vi "save_to_disk.vi"(3 "Retrace":i16[][](array[numeric]), 4 "slice":i32, 5 "write info file?":bool, 6 "error in":errorcluster, 7 "Scan info":string, 8 "Image":i16[][](array[numeric]), 9 "File path":path) -> (0 "error out":errorcluster)   [LabVIEW 2016]
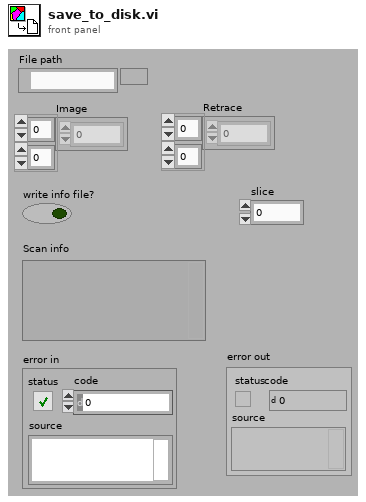
[diagram p1: front panel]
types:
  T1 = cluster{"Rows Per Strip":i32, "Photometric":i32, "Compression Type":i32}
  T2 = typedef "Image Type" = u32
  T3 = typedef "IMAQ Image.ctl" = refnum<image>
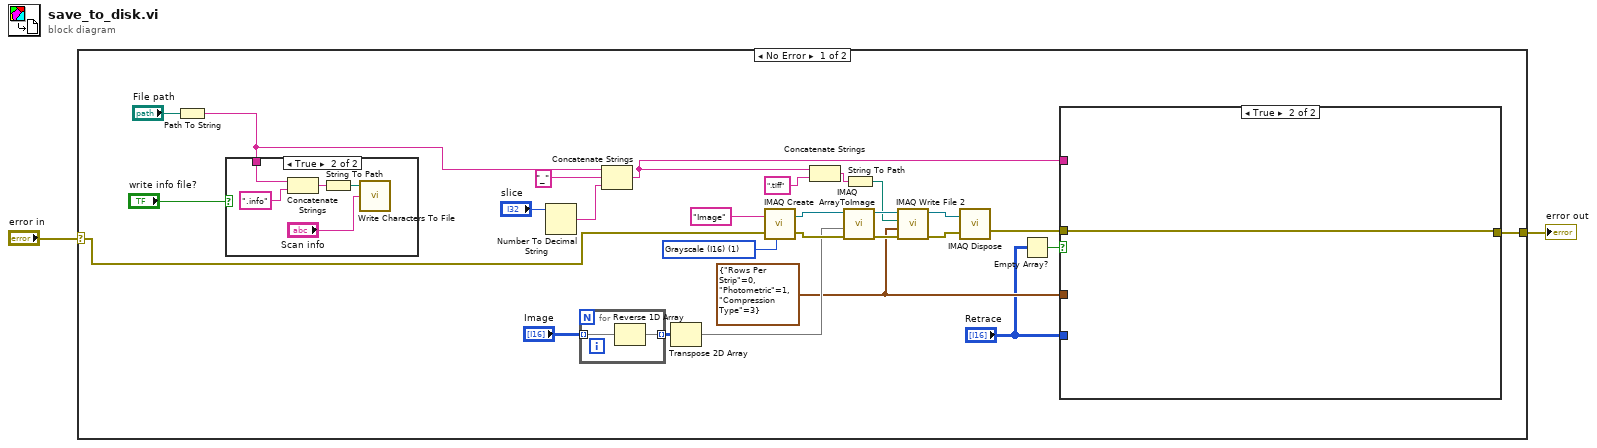
[diagram p0: block diagram]
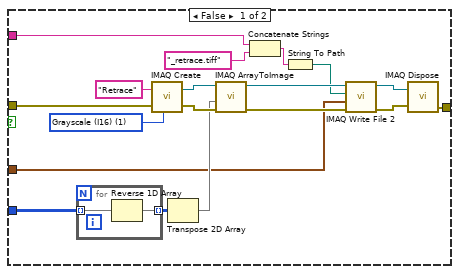
[diagram p2: hidden frame]
diagram:
  n1 = case shown="No Error" "error in" {
    selector: "error in" -> [w5 w58]
    tunnel: [w14 w58] -> w2
    frame No Error {
      w7 = T1 {"Rows Per Strip"=0, "Photometric"=1, "Compression Type"=3} ("TIFF Options")
      w22 = T2 1 items=["Grayscale (U8)", "Grayscale (I16)", "Grayscale (SGL)", "Complex (CSG)", "RGB (U32)", "HSL (U32)", "RGB (U64)", "Grayscale (U16)"] ("Image Type")
      n2 = Path To String(path="File path") -> (string=w12:string)
      n3 = case shown="True" "write info file?" {
        tunnel: w12 -> [_ w52]
        frame False {
        }
        frame True {
          n4 = Concatenate Strings(w52, ".info" ("string")) -> (w53:string)
          n5 = String To Path(string=w53) -> (path=w54:path)
          n6 = call <vilib>:"Write Characters To File.vi"("character string"="Scan info", "file path (dialog if empty)"=w54) -> ()  [unwired: 3 in, 1 out]
        }
      }
      n7 = Number To Decimal String(number="slice") -> (decimal integer string=w10:string)  [unwired: 1 in]
      n8 = for {
        tunnel: "Image" -> [w57] mode=indexing
        tunnel: [w56] -> w19 mode=indexing
        n9 = Reverse 1D Array(array=w57) -> (reversed array=w56:i16[])
      }
      n10 = Concatenate Strings(w12, "_" ("string"), w10) -> (w9:string)
      n11 = Transpose 2D Array(2D array=w19) -> (transposed array=w18:i16[][])
      n12 = call "IMAQ Create"("Image Name"="Image", "Image Type"=w22, "error in (no error)"=w5) -> ("New Image"=w29:T3, "error out"=w27:errorcluster)  [unwired: 2 in]
      n13 = Concatenate Strings(w9, ".tiff" ("string")) -> (w21:string)
      n14 = call "IMAQ ArrayToImage"("error in (no error)"=w27, "Image Pixels (I16)"=w18, "Image"=w29) -> ("error out"=w26:errorcluster, "Image Out"=w25:T3)  [unwired: 7 in]
      n15 = String To Path(string=w21) -> (path=w20:path)
      n16 = call-poly "IMAQ Write File 2"("error in (no error)"=w26, "TIFF Options"=w7, "File Path"=w20, "Image"=w25) -> ("error out"=w23:errorcluster, "Image Out (duplicate)"=w24:T3)  [unwired: 6 in]
      n17 = call "IMAQ Dispose"("Image"=w24, "error in (no error)"=w23) -> ("error out"=w13:errorcluster)  [unwired: 4 in]
      n18 = Empty Array?(array="Retrace") -> (empty?=w4:bool)
      n19 = case shown="True" w4 {
        tunnel: [w37 w50] -> w14
        tunnel: w13 -> [w36 w50]
        tunnel: "Retrace" -> [w34 _]
        tunnel: w9 -> [w32 _]
        tunnel: w7 -> [w30 _]
        frame False {
          w40 = T2 1 items=["Grayscale (U8)", "Grayscale (I16)", "Grayscale (SGL)", "Complex (CSG)", "RGB (U32)", "HSL (U32)", "RGB (U64)", "Grayscale (U16)"] ("Image Type")
          n20 = for {
            tunnel: w34 -> [w49] mode=indexing
            tunnel: [w48] -> w35 mode=indexing
            n21 = Reverse 1D Array(array=w49) -> (reversed array=w48:i16[])
          }
          n22 = call "IMAQ Create"("Image Name"="Retrace", "Image Type"=w40, "error in (no error)"=w36) -> ("New Image"=w39:T3, "error out"=w38:errorcluster)  [unwired: 2 in]
          n23 = Transpose 2D Array(2D array=w35) -> (transposed array=w33:i16[][])
          n24 = call "IMAQ ArrayToImage"("error in (no error)"=w38, "Image Pixels (I16)"=w33, "Image"=w39) -> ("error out"=w47:errorcluster, "Image Out"=w46:T3)  [unwired: 7 in]
          n25 = Concatenate Strings(w32, "_retrace.tiff" ("string")) -> (w43:string)
          n26 = String To Path(string=w43) -> (path=w42:path)
          n27 = call-poly "IMAQ Write File 2"("error in (no error)"=w47, "TIFF Options"=w30, "File Path"=w42, "Image"=w46) -> ("error out"=w44:errorcluster, "Image Out (duplicate)"=w45:T3)  [unwired: 6 in]
          n28 = call "IMAQ Dispose"("Image"=w45, "error in (no error)"=w44) -> ("error out"=w37:errorcluster)  [unwired: 4 in]
        }
        frame True {
        }
      }
    }
    frame Error {
    }
  }
  "error out" <- w2
